vi "Controller Conditioning Vector Test.vi"() -> ()   [LabVIEW 2017]
uses:
  Controller Conditioning Enum.ctl
panel:
  out "Array":cluster{"X":dbl, "Y":dbl}[](array[cluster])
  out "XY Graph":cluster{"X":dbl, "Y":dbl}[](graph)
  in  "stop":bool
  out "output cluster":T1
  in  "X(-1 to 1)":dbl
  in  "Y(-1 to 1)":dbl
  in  "Dead Zone(0 to 1)":dbl
  in  "Enum":T2(ring)
  in  "n^x(Unbounded)":dbl=2.5 format="%#_13g"
  in  "Min Output(0 to 1)":dbl
  in  "Angular Offset\n(-180 to 180 or 0 to 360)":dbl
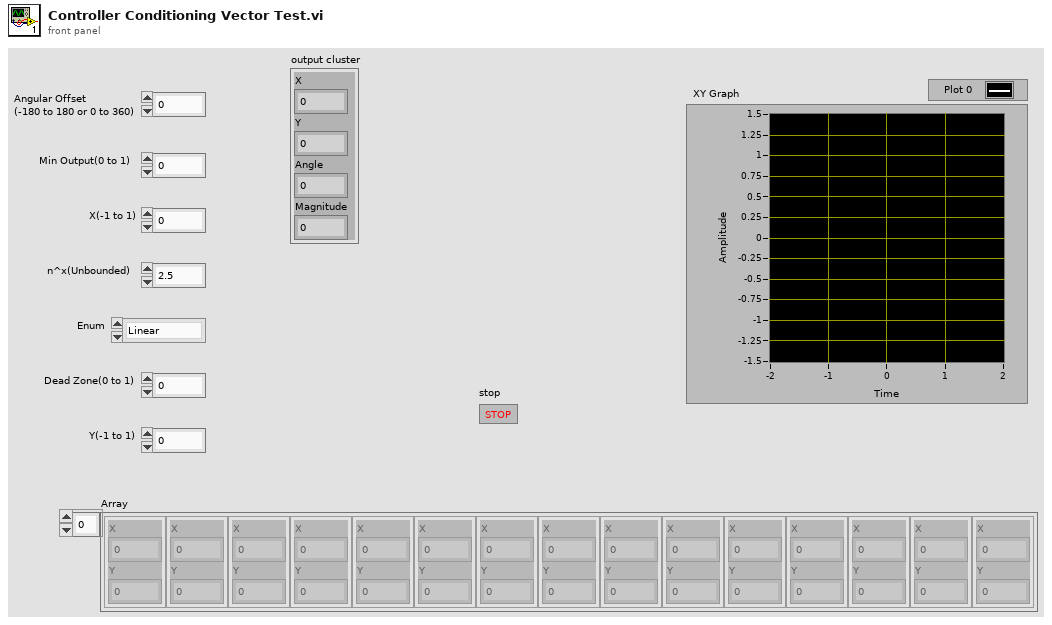
[diagram p1: front panel]
types:
  T1 = cluster{"X":dbl, "Y":dbl, "Angle":dbl, "Magnitude":dbl}
  T2 = enum16{"Linear", "Square  Root", "Square", "n^x"}
  T3 = typedef "Controller Conditioning Enum.ctl" = enum16{"Idle", "Calculate", "Stop"}
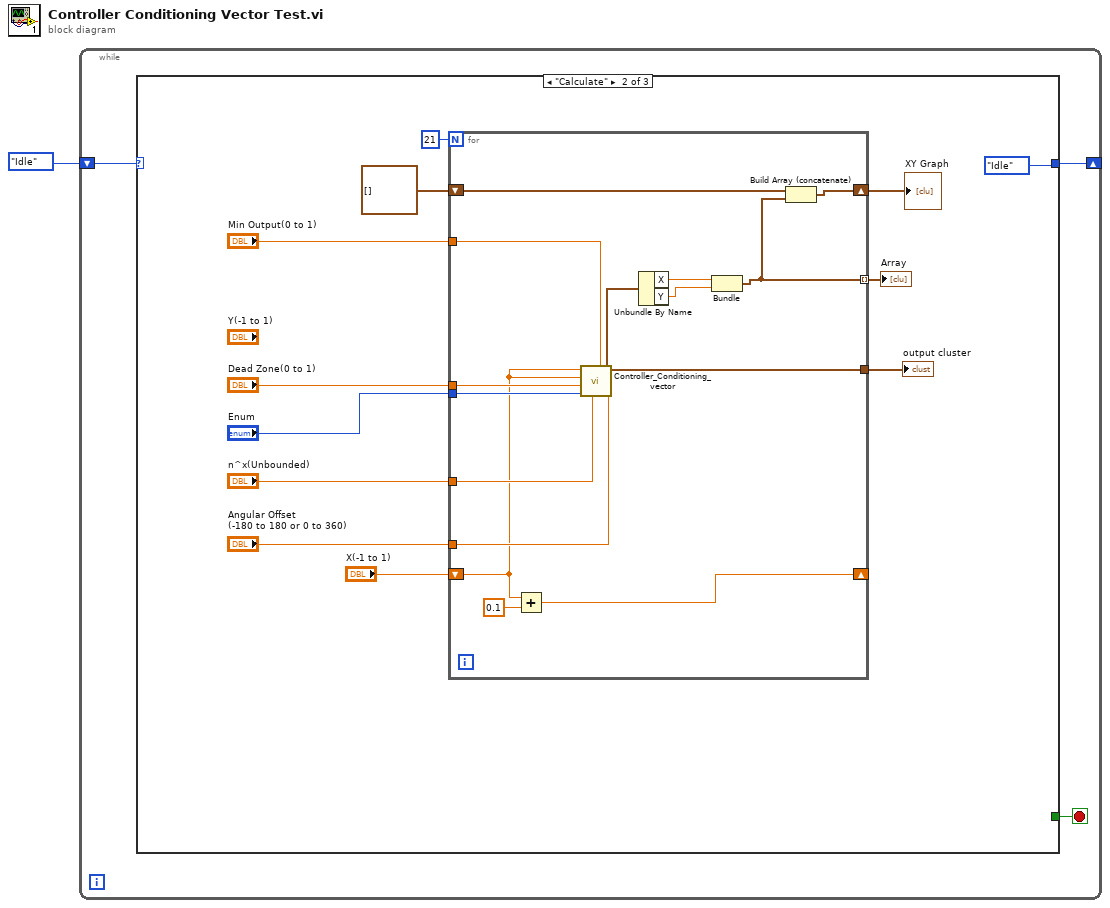
[diagram p0: block diagram]
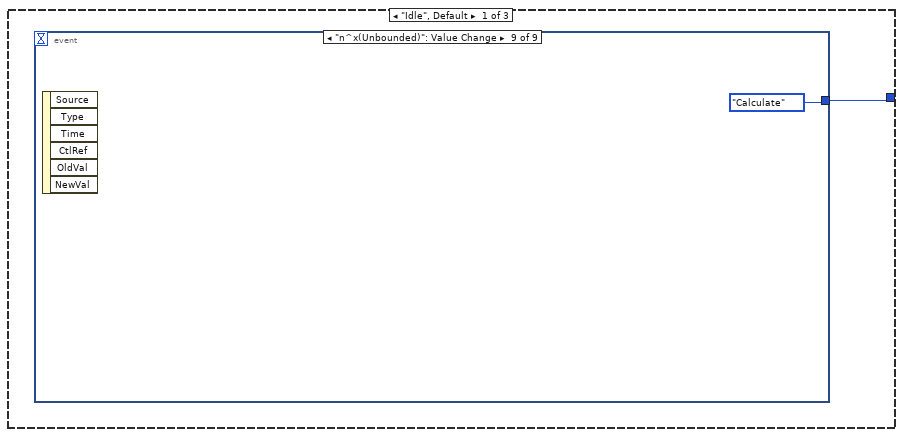
[diagram p2: hidden frame]
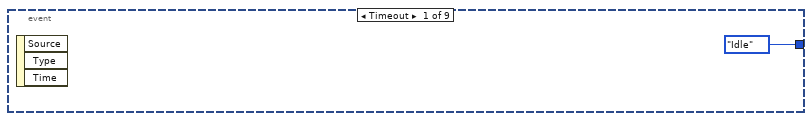
[diagram p3: hidden frame]
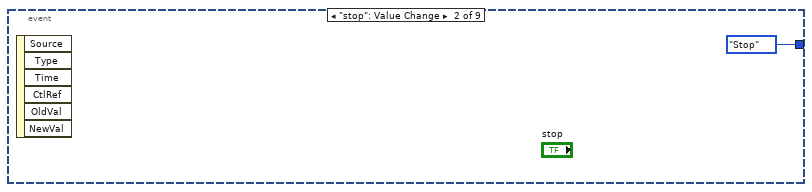
[diagram p4: hidden frame]
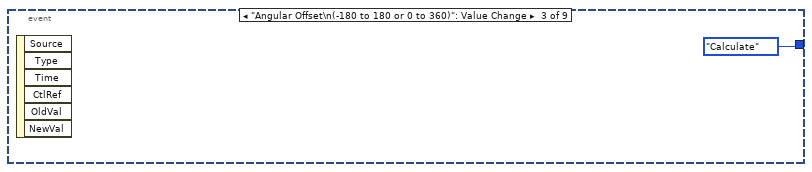
[diagram p5: hidden frame]
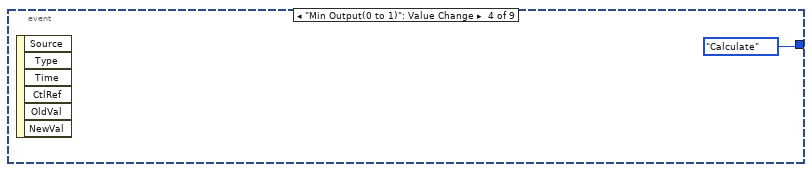
[diagram p6: hidden frame]
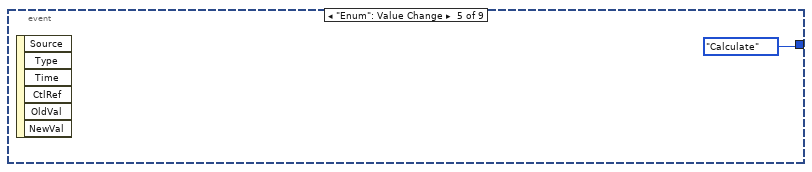
[diagram p7: hidden frame]
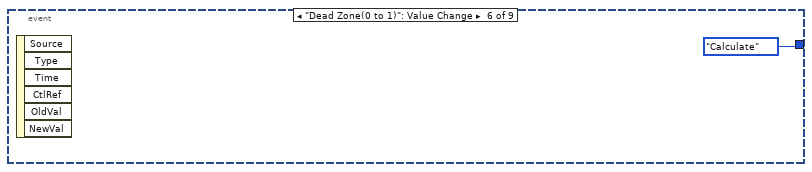
[diagram p8: hidden frame]
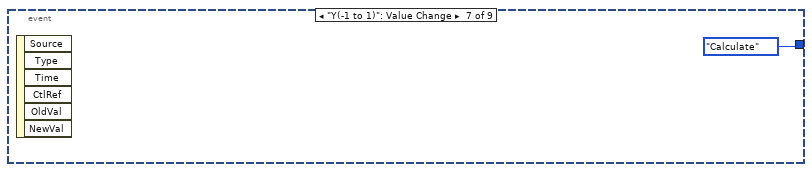
[diagram p9: hidden frame]
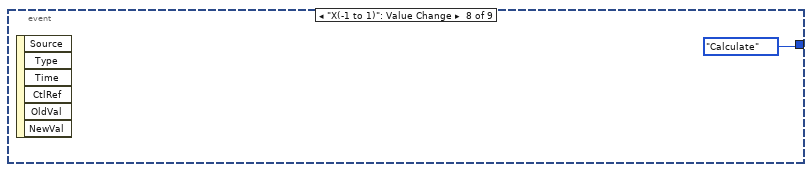
[diagram p10: hidden frame]
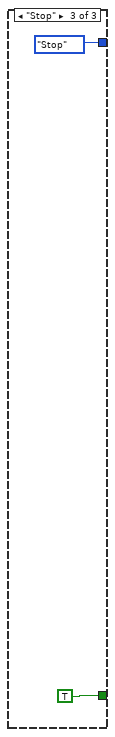
[diagram p11: hidden frame]
diagram:
  n1 = while {
    shift-right: [w2] -> _
    shift-left: Controller_Conditioning_Enum."Idle" ("Enum 2") -> [w4]
    stop <- w3 stop-if-true
    n2 = case shown="\"Calculate\"" w4 {
      tunnel: [_ _ TRUE] -> w3
      tunnel: [w5 Controller_Conditioning_Enum."Idle" ("Enum 2") Controller_Conditioning_Enum."Stop" ("Enum 2")] -> w2
      frame "Idle", Default {
        n3 = event shown="[8] \"n^x(Unbounded)\": Value Change" {
          selector: _ -> [_ _ _ _ _ _ _ _ _]
          dyn-events: _ -> [_ _ _ _ _ _ _ _ _]
          timeout: _ -> [_ _ _ _ _ _ _ _ _]
          tunnel: [Controller_Conditioning_Enum."Idle" ("Enum 2") Controller_Conditioning_Enum."Stop" ("Enum 2") Controller_Conditioning_Enum."Calculate" ("Enum 2") Controller_Conditioning_Enum."Calculate" ("Enum 2") Controller_Conditioning_Enum."Calculate" ("Enum 2") Controller_Conditioning_Enum."Calculate" ("Enum 2") Controller_Conditioning_Enum."Calculate" ("Enum 2") Controller_Conditioning_Enum."Calculate" ("Enum 2") Controller_Conditioning_Enum."Calculate" ("Enum 2")] -> w5
          event Timeout {
            n4 = event-data() -> ()  [unwired: 1 in, 3 out]
          }
          event "stop": Value Change {
            n5 = event-data() -> ()  [unwired: 1 in, 6 out]
          }
          event "Angular Offset\n(-180 to 180 or 0 to 360)": Value Change {
            n6 = event-data() -> ()  [unwired: 1 in, 6 out]
          }
          event "Min Output(0 to 1)": Value Change {
            n7 = event-data() -> ()  [unwired: 1 in, 6 out]
          }
          event "Enum": Value Change {
            n8 = event-data() -> ()  [unwired: 1 in, 6 out]
          }
          event "Dead Zone(0 to 1)": Value Change {
            n9 = event-data() -> ()  [unwired: 1 in, 6 out]
          }
          event "Y(-1 to 1)": Value Change {
            n10 = event-data() -> ()  [unwired: 1 in, 6 out]
          }
          event "X(-1 to 1)": Value Change {
            n11 = event-data() -> ()  [unwired: 1 in, 6 out]
          }
          event "n^x(Unbounded)": Value Change {
            n12 = event-data() -> ()  [unwired: 1 in, 6 out]
          }
        }
      }
      frame "Calculate" {
        n13 = for {
          N: 21 -> [_]
          tunnel: "Angular Offset\n(-180 to 180 or 0 to 360)" -> [w40]
          tunnel: "Min Output(0 to 1)" -> [w39]
          tunnel: "n^x(Unbounded)" -> [w38]
          tunnel: "Enum" -> [w37]
          tunnel: "Dead Zone(0 to 1)" -> [w36]
          tunnel: [w35] -> w20
          shift-right: [w31] -> w18
          shift-left: cluster{"X":dbl, "Y":dbl}[] [] ("XY Graph") -> [w32]
          shift-right: [w29] -> _
          shift-left: "X(-1 to 1)" -> [w28]
          tunnel: [w27] -> w15 mode=indexing
          n14 = Add(x=w28, y=0.1) -> (x+y=w29:dbl)
          n15 = call "Controller_Conditioning_vector.vi"("Angular Offset\n(-180 to 180 or 0 to 360)"=w40, "Min Output(0 to 1)"=w39, "n^x(Unbounded)"=w38, "Enum"=w37, "Dead Zone(0 to 1)"=w36, "Y(-1 to 1)"=w28, "X(-1 to 1)"=w28) -> ("output cluster"=w35:T1)  [unwired: 4 in]
          n16 = Unbundle By Name(w35) -> ("X"=w34:dbl, "Y"=w33:dbl)
          n17 = Bundle("X"=w34, "Y"=w33) -> (w27:cluster{"X":dbl, "Y":dbl})  [unwired: 1 in]
          n18 = Build Array (concatenate)(w32, w27) -> (w31:cluster{"X":dbl, "Y":dbl}[])
        }
        "output cluster" <- w20
        "XY Graph" <- w18
        "Array" <- w15
      }
      frame "Stop" {
      }
    }
  }
